vi "LMTD.vi"(6 "Tube Cold Temp (K)":dbl, 9 "Tube Hot Temp (K)":dbl, 10 "Shell Hot Temp (K)":dbl, 11 "Shell Cold Temperature (K)":dbl) -> (3 "LMTD (K)":dbl)   [LabVIEW 2019]
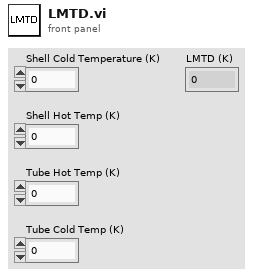
[diagram p1: front panel]
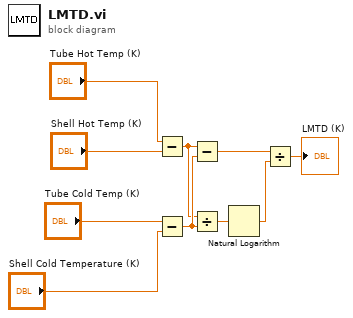
[diagram p0: block diagram]
diagram:
  n1 = Subtract(x="Tube Hot Temp (K)", y="Shell Hot Temp (K)") -> (x-y=w5:dbl)
  n2 = Subtract(x="Tube Cold Temp (K)", y="Shell Cold Temperature (K)") -> (x-y=w6:dbl)
  n3 = Subtract(x=w5, y=w6) -> (x-y=w8:dbl)
  n4 = Divide(x=w5, y=w6) -> (x/y=w7:dbl)
  n5 = Natural Logarithm(1:w7) -> (0:w9:dbl)
  n6 = Divide(x=w8, y=w9) -> (x/y=→"LMTD (K)":dbl)
